vi "global.vi"() -> ()   [LabVIEW 2016]
panel:
  out "postcharge log file path":path
  out "predischarge log file path":path
  out "discharge state log file path":path
  out "charge state log file path":path
  out "dc resistance log file path":path
  out "raw data log file path":path
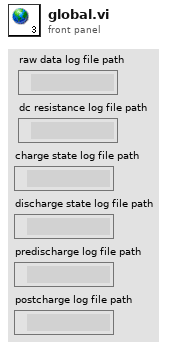
[diagram p1: front panel]
diagram:
